vi "335 set Temp(SubVI).vi"(6 "Input (0:A)":u16(ring)=1 items=["A", "B"], 7 "Output (1:1)":u16(ring)=1 items=["1"=1, "2"=2], 8 "error in (no error)":errorcluster, 9 "Rate":dbl, 10 "Temperature":dbl, 11 "VISA Refnum in":refnum<visa-resource-name>) -> (0 "error out":errorcluster, 3 "VISA resource name out":refnum<visa-resource-name>)   [LabVIEW 2019, in "SubVI.lvlib"]
uses:
  SubVI.lvlib
  lib/Lake Shore 335/Lake Shore 335.lvlib
panel:
  out "Sensor Data":dbl format="%.4f"
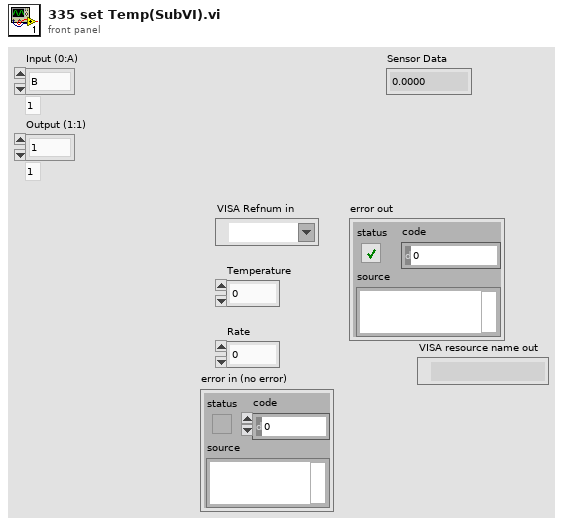
[diagram p1: front panel]
types:
  T1 = typedef "Semaphore RefNum" = refnum<k1>
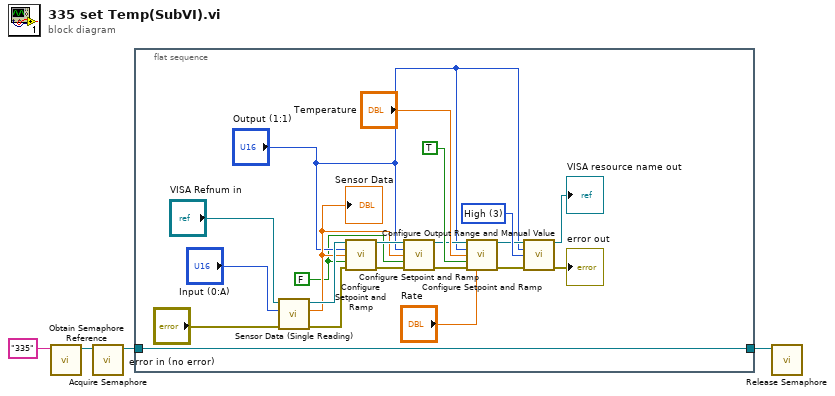
[diagram p0: block diagram]
diagram:
  n1 = call <vilib>:"Obtain Semaphore Reference.vi"("name (unnamed)"="335") -> ("semaphore"=w3:T1)  [unwired: 4 in, 2 out]
  n2 = call <vilib>:"Acquire Semaphore.vi"("semaphore"=w3) -> ("semaphore out"=w2:T1)  [unwired: 4 in, 2 out]
  n3 = flat-sequence {
    tunnel: w2 -> [w13]
    tunnel: [w13] -> w1
    frame #0 {
      w24 = u16 3 items=["Off", "Low (On)", "Medium", "High"] ("Range (0:Off)")
      w5 = FALSE ("Enable Setpoint Ramping (F: Off)")
      n4 = call "Sensor Data (Single Reading).vi"("error in (no error)"="error in (no error)", "Input (0:A)"="Input (0:A)", "VISA resource name"="VISA Refnum in") -> ("error out"=w15:errorcluster, "Sensor Data"=w7:dbl, "VISA resource name out"=w19:refnum<visa-resource-name>)  [unwired: 6 in]
      "Sensor Data" <- w7
      n5 = call "Configure Setpoint and Ramp.vi"("VISA resource name"=w19, "Output's Control Loop (1:1)"="Output (1:1)", "Setpoint (0.0000)"=w7, "Enable Setpoint Ramping (F: Off)"=w5, "error in (no error)"=w15) -> ("VISA resource name out"=w9:refnum<visa-resource-name>, "error out"=w11:errorcluster)  [unwired: 9 in]
      n6 = call "Configure Setpoint and Ramp.vi"("VISA resource name"=w9, "Output's Control Loop (1:1)"="Output (1:1)", "Setpoint (0.0000)"=w7, "Enable Setpoint Ramping (F: Off)"=w5, "error in (no error)"=w11) -> ("VISA resource name out"=w8:refnum<visa-resource-name>, "error out"=w10:errorcluster)  [unwired: 9 in]
      n7 = call "Configure Setpoint and Ramp.vi"("VISA resource name"=w8, "Output's Control Loop (1:1)"="Output (1:1)", "Setpoint (0.0000)"="Temperature", "Enable Setpoint Ramping (F: Off)"=TRUE, "error in (no error)"=w10, "Ramp Rate (0.0)"="Rate") -> ("VISA resource name out"=w23:refnum<visa-resource-name>, "error out"=w14:errorcluster)  [unwired: 8 in]
      n8 = call "Configure Output Range and Manual Value.vi"("VISA resource name"=w23, "Heater Output (1:1)"="Output (1:1)", "Range (0:Off)"=w24, "error in (no error)"=w14) -> ("VISA resource name out"=→"VISA resource name out":refnum<visa-resource-name>, "error out"=→"error out":errorcluster)  [unwired: 10 in]
    }
  }
  n9 = call <vilib>:"Release Semaphore.vi"("semaphore"=w1) -> ()  [unwired: 5 in, 2 out]
